vi "strict.TestToReportEntry.vi"(8 "error in (no error)":errorcluster, 9 "Asserts (aka. Test Cases)":T4[](array[typedef]), 10 "Node (aka. Test Suite)":T5) -> (0 "error out":errorcluster, 1 "testcases":T1[](array[typedef]), 2 "testsuite":T2)   [LabVIEW 2013, in "strict-JUnit.lvclass"]
uses:
  strict-JUnit.lvclass
  <vilib>/addons/_JKI Toolkits/Caraya/classes/Test Result/Test Node.ctl
  <vilib>/addons/_JKI Toolkits/Caraya/classes/Test Result/Test Registration Data.ctl
  <vilib>/addons/_JKI Toolkits/Caraya/classes/Test Result/Assert Event Data.ctl
  <vilib>/addons/_JKI Toolkits/Caraya/classes/Test Report.JUnit/testsuite -- cluster.ctl
  <vilib>/addons/_JKI Toolkits/Caraya/classes/Test Report.JUnit/property -- cluster.ctl
  <vilib>/addons/_JKI Toolkits/Caraya/classes/Test Report.JUnit/testcase -- cluster.ctl
  <vilib>/addons/_JKI Toolkits/Caraya/classes/Test Report.JUnit/Test Report.JUnit.lvclass
  <vilib>/addons/_JKI Toolkits/Caraya/classes/Test Result/Test Result.lvclass
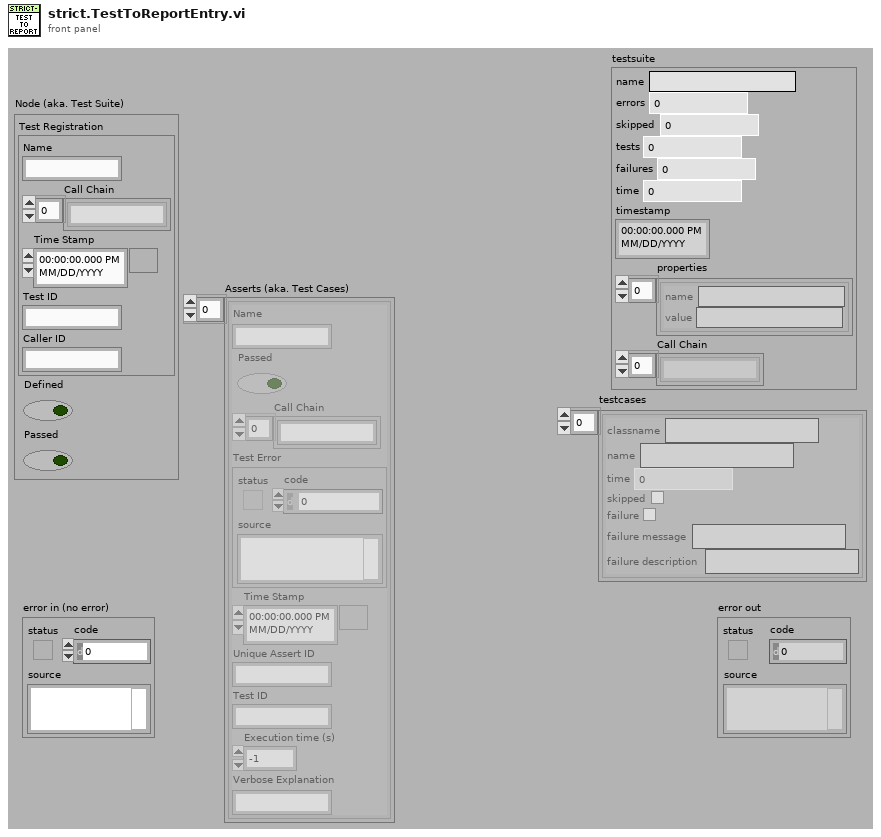
[diagram p1: front panel]
types:
  T1 = typedef "Caraya.lvlib/Test Report.JUnit.lvclass/testcase -- cluster.ctl" = cluster{"classname":string, "name":string, "time":dbl, "skipped":bool, "failure":bool, "failure message":string, "failure description":string}
  T2 = typedef "Caraya.lvlib/Test Report.JUnit.lvclass/testsuite -- cluster.ctl" = cluster{"name":string, "errors":u32, "skipped":u32, "tests":u32, "failures":u32, "time":dbl, "timestamp":timestamp, "properties":T3[], "Call Chain":string[]}
  T3 = typedef "Caraya.lvlib/Test Report.JUnit.lvclass/property -- cluster.ctl" = cluster{"name":string, "value":string}
  T4 = typedef "Caraya.lvlib/Test Result.lvclass/Assert Event Data.ctl" = cluster{"Name":string, "Passed":bool, "Call Chain":string[], "Test Error":errorcluster, "Time Stamp":timestamp, "Unique Assert ID":string, "Test ID":string, "Execution time (s)":dbl, "Verbose Explanation":string}
  T5 = typedef "Caraya.lvlib/Test Result.lvclass/Test Node.ctl" = cluster{"Test Registration":T6, "Defined":bool, "Passed":bool}
  T6 = typedef "Caraya.lvlib/Test Result.lvclass/Test Registration Data.ctl" = cluster{"Name":string, "Call Chain":string[], "Time Stamp":timestamp, "Test ID":string, "Caller ID":string}
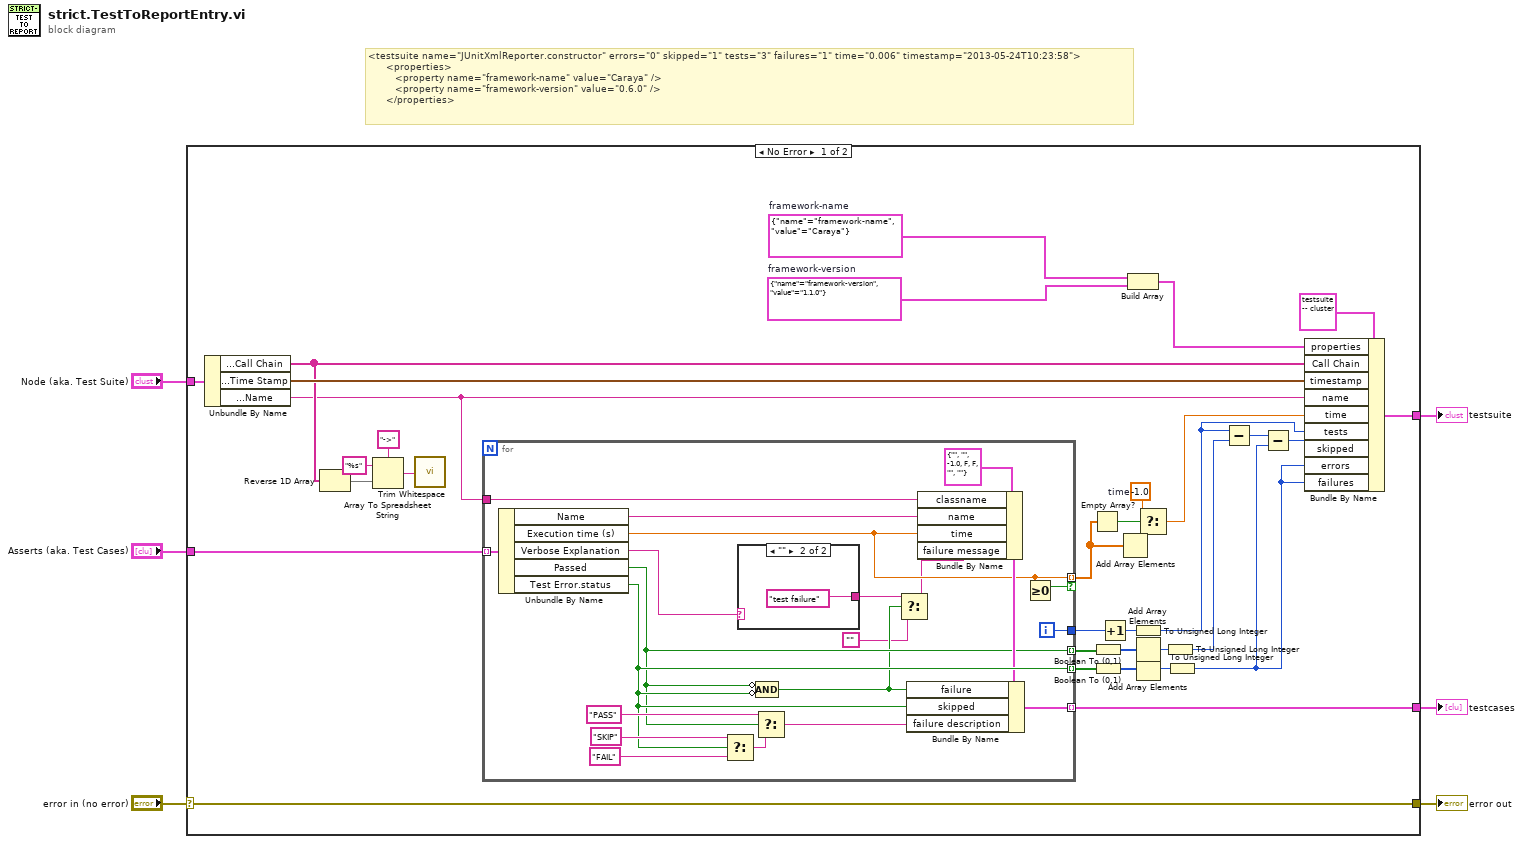
[diagram p0: block diagram]
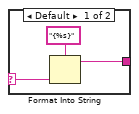
[diagram p2: hidden frame]
diagram:
  # "<testsuite name=\"JUnitXmlReporter.constructor\" errors=\"0\" skipped=\"1\" tests=\"3\" failures=\"1\" time=\"0.006\" timestamp=\"2013-05-24T10:23:58\">\n      <properties>\n         <property name=\"framework-name\" value=\"Caraya\" />\n         <property name=\"framework-version\" value=\"0.6.0\" />\n      </properties>"
  n1 = case shown="No Error" "error in (no error)" {
    selector: "error in (no error)" -> [w39 w66]
    tunnel: [w39 w66] -> w5
    tunnel: "Node (aka. Test Suite)" -> [w40 _]
    tunnel: "Asserts (aka. Test Cases)" -> [w38 _]
    tunnel: [w33 _] -> w2
    tunnel: [w32 _] -> w1
    frame No Error {
      w7 = T3 {"name"="framework-version", "value"="1.1.0"}  # framework-version
      w16 = T3 {"name"="framework-name", "value"="Caraya"}  # framework-name
      w23 = -1.0  # time
      n2 = Unbundle By Name(w40) -> ("Test Registration.Call Chain"=w13:string[], "Test Registration.Time Stamp"=w20:timestamp, "Test Registration.Name"=w8:string)
      n3 = Reverse 1D Array(array=w13) -> (reversed array=w12:string[])
      n4 = Array To Spreadsheet String(delimiter (Tab)="->", array=w12, 3:"%s" ("format string")) -> (spreadsheet string=w9:string)
      n5 = call <vilib>:"Trim Whitespace.vi"("string"=w9) -> ()  [unwired: 1 in, 1 out]
      n6 = for {
        tunnel: w38 -> [w61] mode=indexing
        tunnel: [w46] -> w37 mode=indexing
        tunnel: [w53] -> w29 mode=indexing
        tunnel: w8 -> [w51]
        tunnel: [w60] -> w32 mode=indexing
        tunnel: [w47] -> w25 mode=indexing if=w55
        tunnel: [w52] -> w21
        i -> [w52]
        n7 = Unbundle By Name(w61) -> ("Name"=w48:string, "Execution time (s)"=w47:dbl, "Verbose Explanation"=w41:string, "Passed"=w46:bool, "Test Error.status"=w53:bool)
        n8 = Select(t="SKIP" ("failure message"), s=w53, f="FAIL" ("failure message")) -> (s? t:f=w58:string)
        n9 = case shown="\"\"" w41 {
          selector: w41 -> [w62 _]
          tunnel: [w63 "test failure" ("failure message")] -> w42
          frame Default {
            n10 = Format Into String(format string="{%s}", w62) -> (resulting string=w63:string)  [unwired: 2 in, 1 out]
          }
          frame "" {
          }
        }
        n11 = Compound Arithmetic op=AND(invert w46, invert w53) -> (w45:bool)
        n12 = Select(t="PASS" ("failure message"), s=w46, f=w58) -> (s? t:f=w54:string)
        n13 = Select(t=w42, s=w45, f="") -> (s? t:f=w43:string)
        n14 = Bundle By Name(cluster=T1 {"classname"="", "name"="", "time"=-1.0, "skipped"=FALSE, "failure"=FALSE, "failure message"="", "failure description"=""} ("testcase"), "classname"=w51, "name"=w48, "time"=w47, "failure message"=w43) -> (w49:T1)
        n15 = Bundle By Name(cluster=w49, "failure"=w45, "skipped"=w53, "failure description"=w54) -> (w60:T1)
        n16 = Greater Or Equal To 0?(x=w47) -> (x >= 0?=w55:bool)
      }
      n17 = Empty Array?(array=w25) -> (empty?=w24:bool)
      n18 = Boolean To (0,1)(Boolean=w37) -> (0, 1=w36:i16[])
      n19 = Boolean To (0,1)(Boolean=w29) -> (0, 1=w30:i16[])
      n20 = Increment(x=w21) -> (x+1=w17:i32)
      n21 = Add Array Elements(numeric array=w25) -> (sum=w22:dbl)
      n22 = Build Array(w16, w7) -> (w15:T3[])
      n23 = To Unsigned Long Integer(number=w17) -> (unsigned 32bit integer=w14:u32)
      n24 = Add Array Elements(numeric array=w36) -> (sum=w31:i16)
      n25 = Add Array Elements(numeric array=w30) -> (sum=w28:i16)
      n26 = Select(t=w23, s=w24, f=w22) -> (s? t:f=w19:dbl)
      n27 = To Unsigned Long Integer(number=w31) -> (unsigned 32bit integer=w27:u32)
      n28 = To Unsigned Long Integer(number=w28) -> (unsigned 32bit integer=w26:u32)
      n29 = Subtract(x=w14, y=w27) -> (x-y=w35:u32)
      n30 = Subtract(x=w35, y=w26) -> (x-y=w34:u32)
      n31 = Bundle By Name(cluster=T2 {"name"="", "errors"=0, "skipped"=0, "tests"=0, "failures"=0, "time"=-1.0, "timestamp"=timestamp(0 s since 1904-01-01), "properties"=[], "Call Chain"=[]} ("testsuite"), "properties"=w15, "Call Chain"=w13, "timestamp"=w20, "name"=w8, "time"=w19, "tests"=w14, "skipped"=w34, "errors"=w26, "failures"=w26) -> (w33:T2)
    }
    frame Error {
    }
  }
  "error out" <- w5
  "testsuite" <- w2
  "testcases" <- w1
